vi "toDouble.vi"(8 "error in (no error)":errorcluster, 11 "Value":variant) -> (0 "error out":errorcluster, 3 "type":dbl)   [LabVIEW 2018, in "Account History.lvclass"]
uses:
  Account History.lvclass
  <vilib>/addons/database/NI_Database_API.lvlib
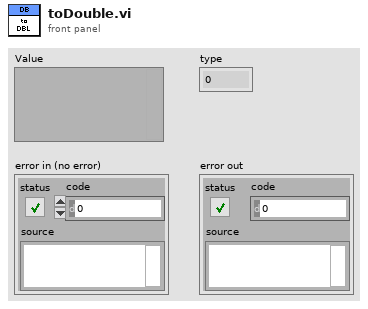
[diagram p1: front panel]
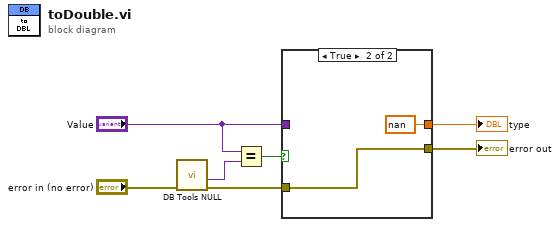
[diagram p0: block diagram]
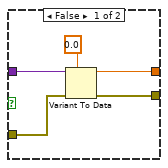
[diagram p2: hidden frame]
diagram:
  n1 = call <vilib>:"DB Tools NULL.vi"("error in (no error)"="error in (no error)") -> ("error out"=w5:errorcluster, "NULL"=w6:variant)  [unwired: 9 in]
  n2 = Equal?(x="Value", y=w6) -> (x = y?=w7:bool)
  n3 = case shown="True" w7 {
    tunnel: [w12 w13] -> w1
    tunnel: [w11 nan ("type")] -> w2
    tunnel: "Value" -> [w9 _]
    tunnel: w5 -> [w8 w13]
    frame False {
      n4 = Variant To Data(error in=w8, type=0.0, Variant=w9) -> (data=w11:dbl, error out=w12:errorcluster)
    }
    frame True {
    }
  }
  "type" <- w2
  "error out" <- w1
